vi "Add Resonance.vi"(8 "error in (no error)":errorcluster, 9 "Y":dbl, 10 "X":dbl, 11 "Resonance Detector in":refnum<class "Resonance Detector.lvclass">) -> (0 "error out":errorcluster, 3 "Resonance Detector out":refnum<class "Resonance Detector.lvclass">)   [LabVIEW 2019, in "Resonance Detector.lvclass"]
uses:
  Resonance Detector.lvclass
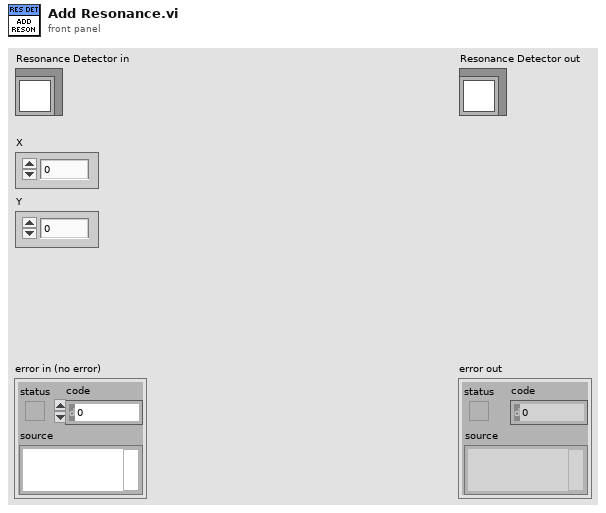
[diagram p1: front panel]
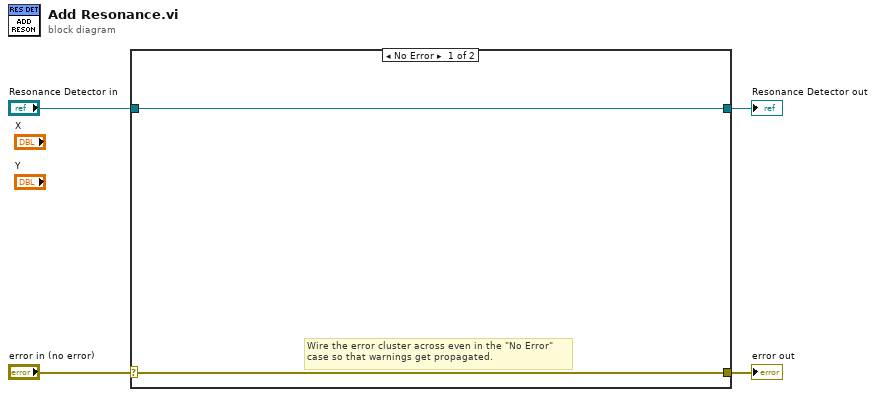
[diagram p0: block diagram]
diagram:
  n1 = case shown="No Error" "error in (no error)" {
    selector: "error in (no error)" -> [w5 w8]
    tunnel: [w5 w8] -> w3
    tunnel: [w6 w7] -> w1
    tunnel: "Resonance Detector in" -> [w6 w7]
    frame No Error {
      # "Wire the error cluster across even in the \"No Error\"\ncase so that warnings get propagated."
    }
    frame Error {
    }
  }
  "error out" <- w3
  "Resonance Detector out" <- w1
